vi "main.vi"() -> ()   [LabVIEW 2018]
uses:
  project/type defs/test keypad luster.ctl
  <vilib>/Instr/_visa.llb/VISA Flush IO Buffer Mask.ctl
  <vilib>/Instr/_visa.llb/VISA Configure Serial Port (Instr).vi
  <vilib>/NI/Modbus Library/API/Wrapper/Create Serial Master.vi
  global variables/offset.vi
  type defs/Pelco_D_cmd.vi
  <vilib>/NI/Modbus Library/API/Master/Modbus Master.lvclass
  <vilib>/NI/Modbus Library/API/Wrapper/API Main.lvlib
panel:
  out "Remote TILT":dbl format="%#_6f"
  out "Remote PAN":dbl format="%#_6f"
  in  "Client Closed":string="The client VI closed the connection."
  out "tic":u32
  out "Reset status":bool
  in  "enable":bool=TRUE
  out "tilt":dbl
  out "pan":dbl
  in  "pan_right_limit(-10) 2":dbl=-20.0
  in  "pan left_limit(20) 2":dbl=20.0
  in  "tilt_down_limit(-10)":dbl=-10.0
  in  "tilt_up_limit(20)":dbl=20.0
  in  "delta tilt/sec":dbl=0.1 format="%#.13f"
  in  "delta pan/sec":dbl=0.1 format="%#.13f"
  out "launcher.compass":dbl format="%.1f"
  out "launcher.tilt":dbl format="%.1f"
  out "launcher.pan":dbl format="%.1f"
  out "magnification":string
  in  "get magnification":bool
  in  "cam default":bool
  out "Lancher's Parameters":i16[](array[numeric])
  in  "reset":bool
  out "Sync Status":bool
  out "keypad cmd":string
  out "CAM.tilt":dbl format="%#.2g"
  out "Cam,pan":dbl format="%.2f"
  out "cmd from keypad":string[](array[string])
  out "ressponse tilt":string
  in  "read tilt":bool
  out "ressponse pan":string
  in  "read pan":bool
  in  "close com":bool
  in  "open com":bool
  in  "stop":bool
  in  "VISA resource name":refnum<visa-resource-name>="COM6"
  # "Launcher"
  # "Camera"
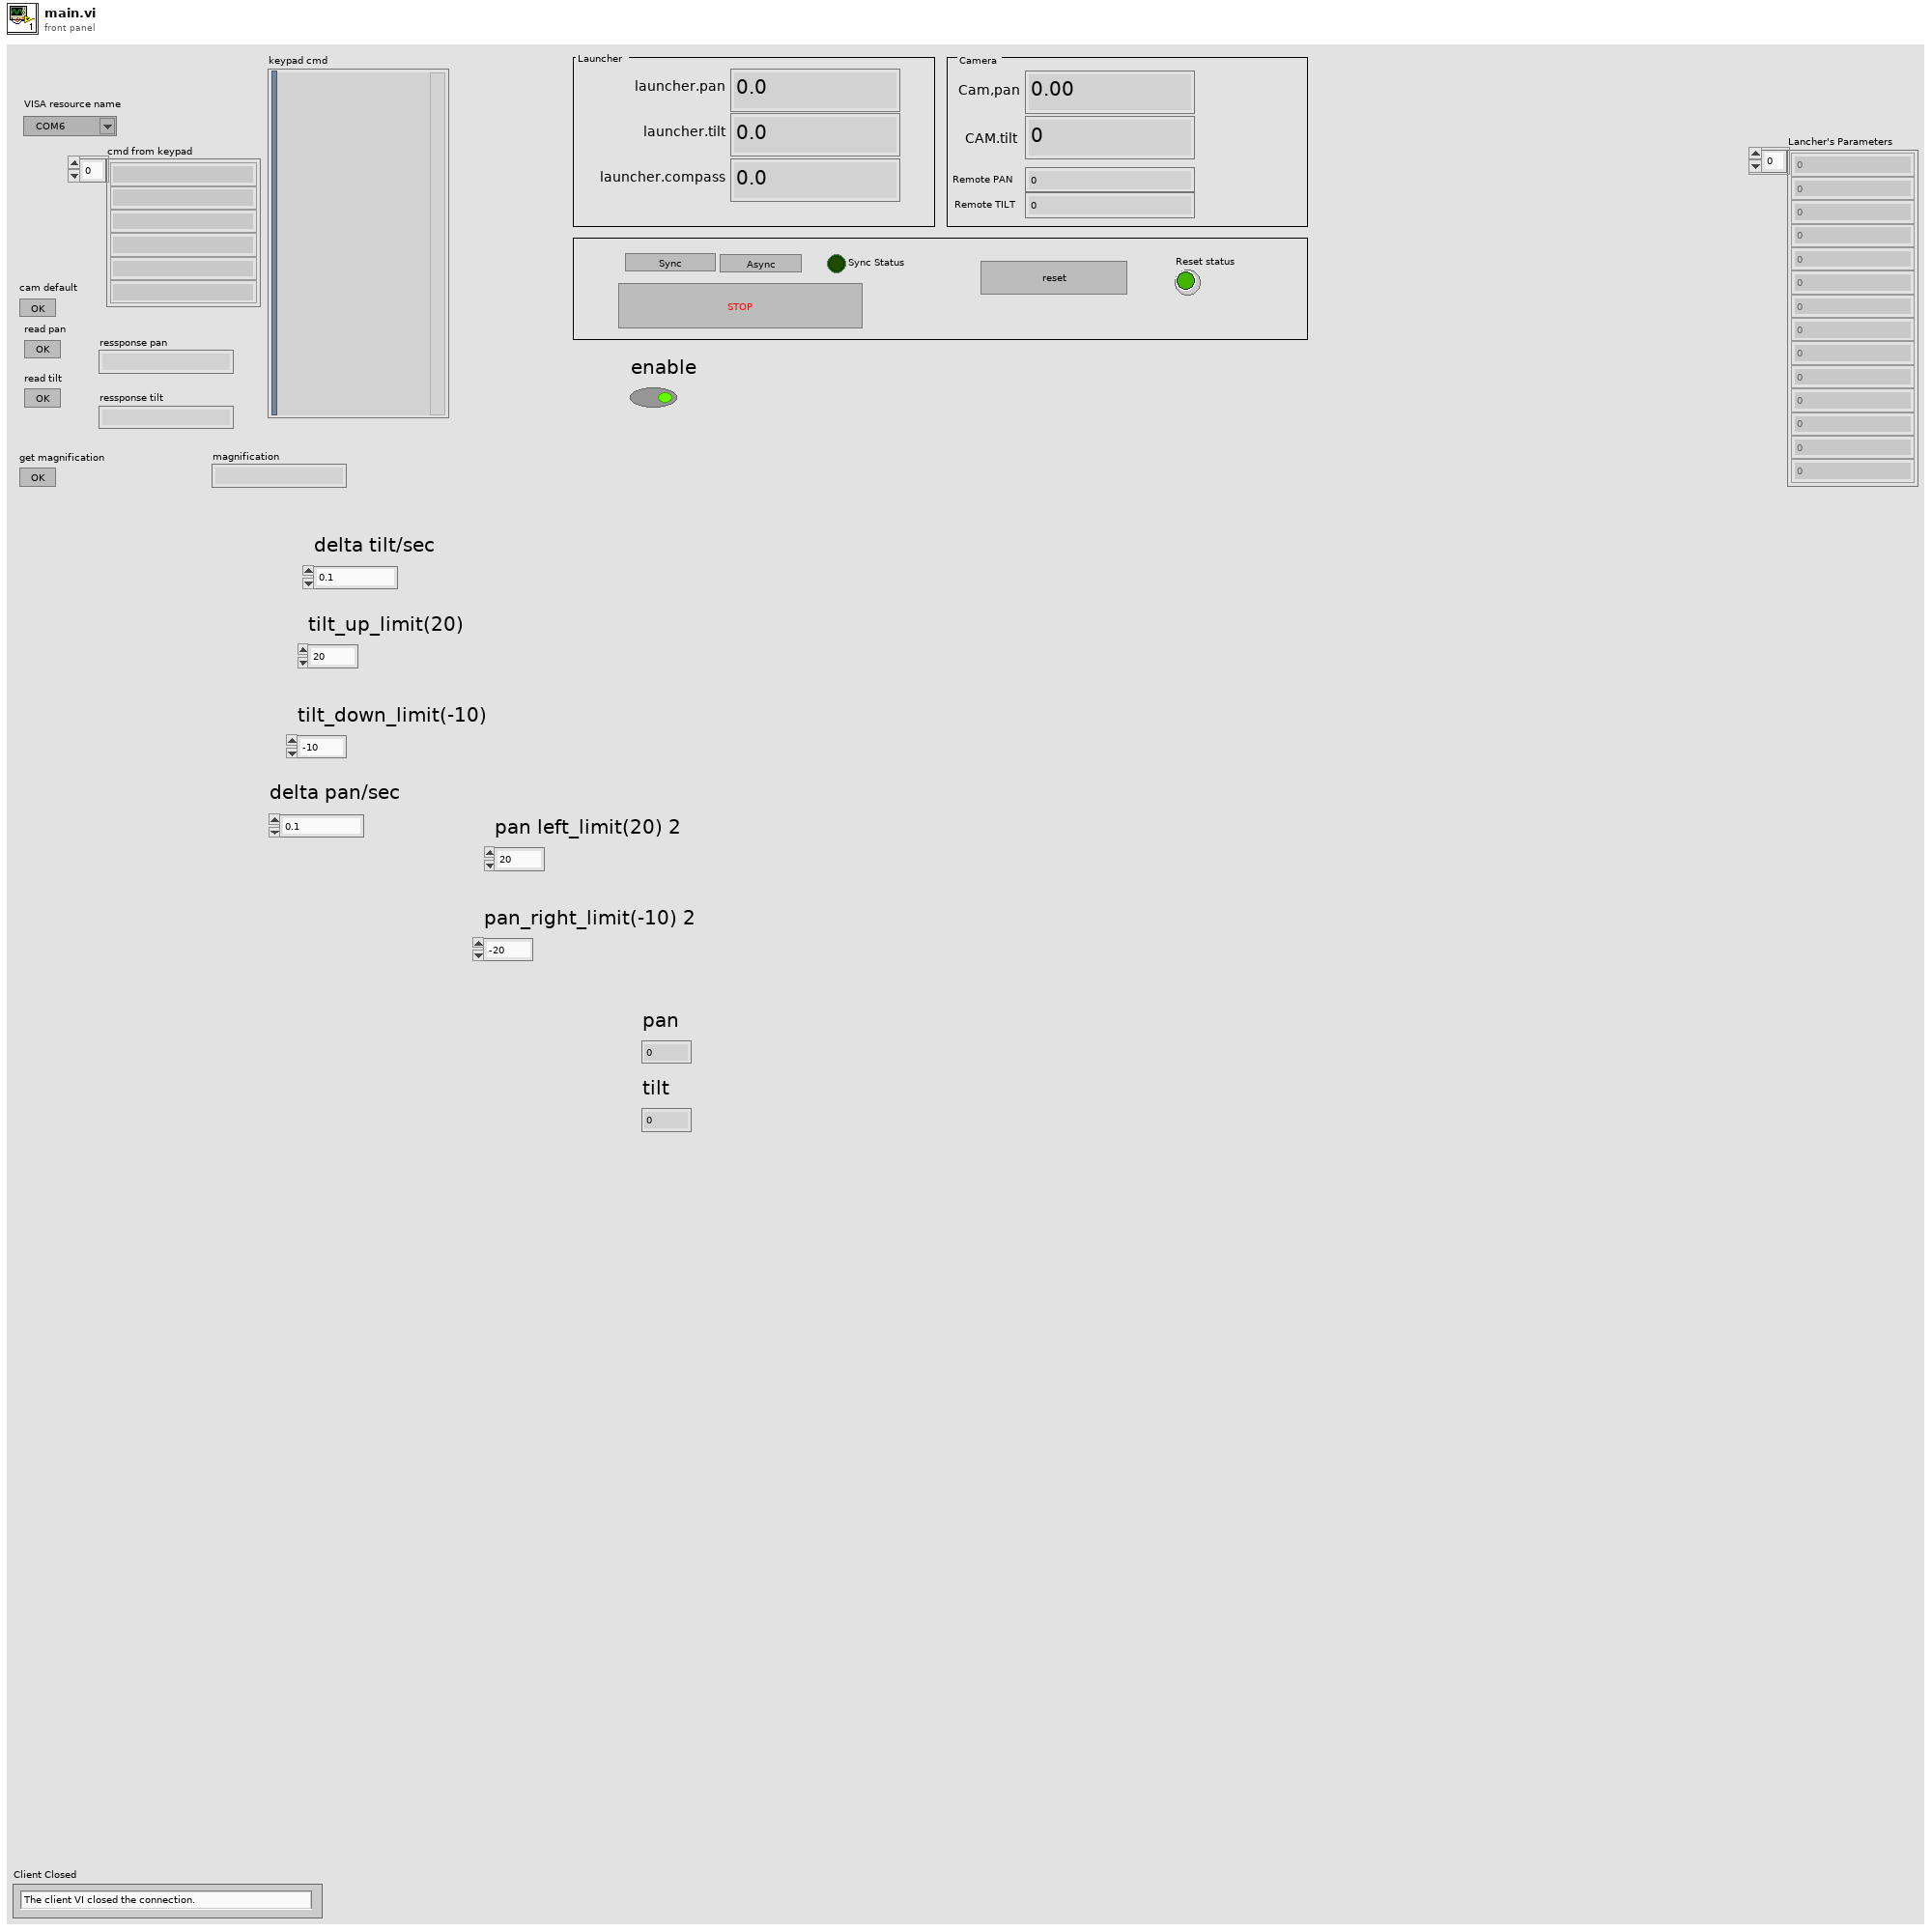
[diagram p1: front panel]
types:
  T1 = cluster{"launcher_pan":i16, "launcher_tilt":i16, "launcher_pan_leftLimit":i16, "launcher_pan_rightLimit":i16, "launcher_tilt_downLimit":i16, "launcher_tilt_upLimit":i16, "launcher_PLClink":i16, "launcher_PLCstatus":i16, "CAM_pan":i16, "CAM_tilt":i16}
  T2 = cluster{"VISA resource name":refnum<visa-resource-name>}
  T3 = typedef "test keypad luster.ctl" = cluster{"cmd":string, "keypad cmd":variant}
  T4 = cluster{"quit":refnum<user-event>, "read tilt":refnum<user-event>, "read pan":refnum<user-event>}
  T5 = typedef "VISA Flush IO Buffer Mask.ctl" = u16
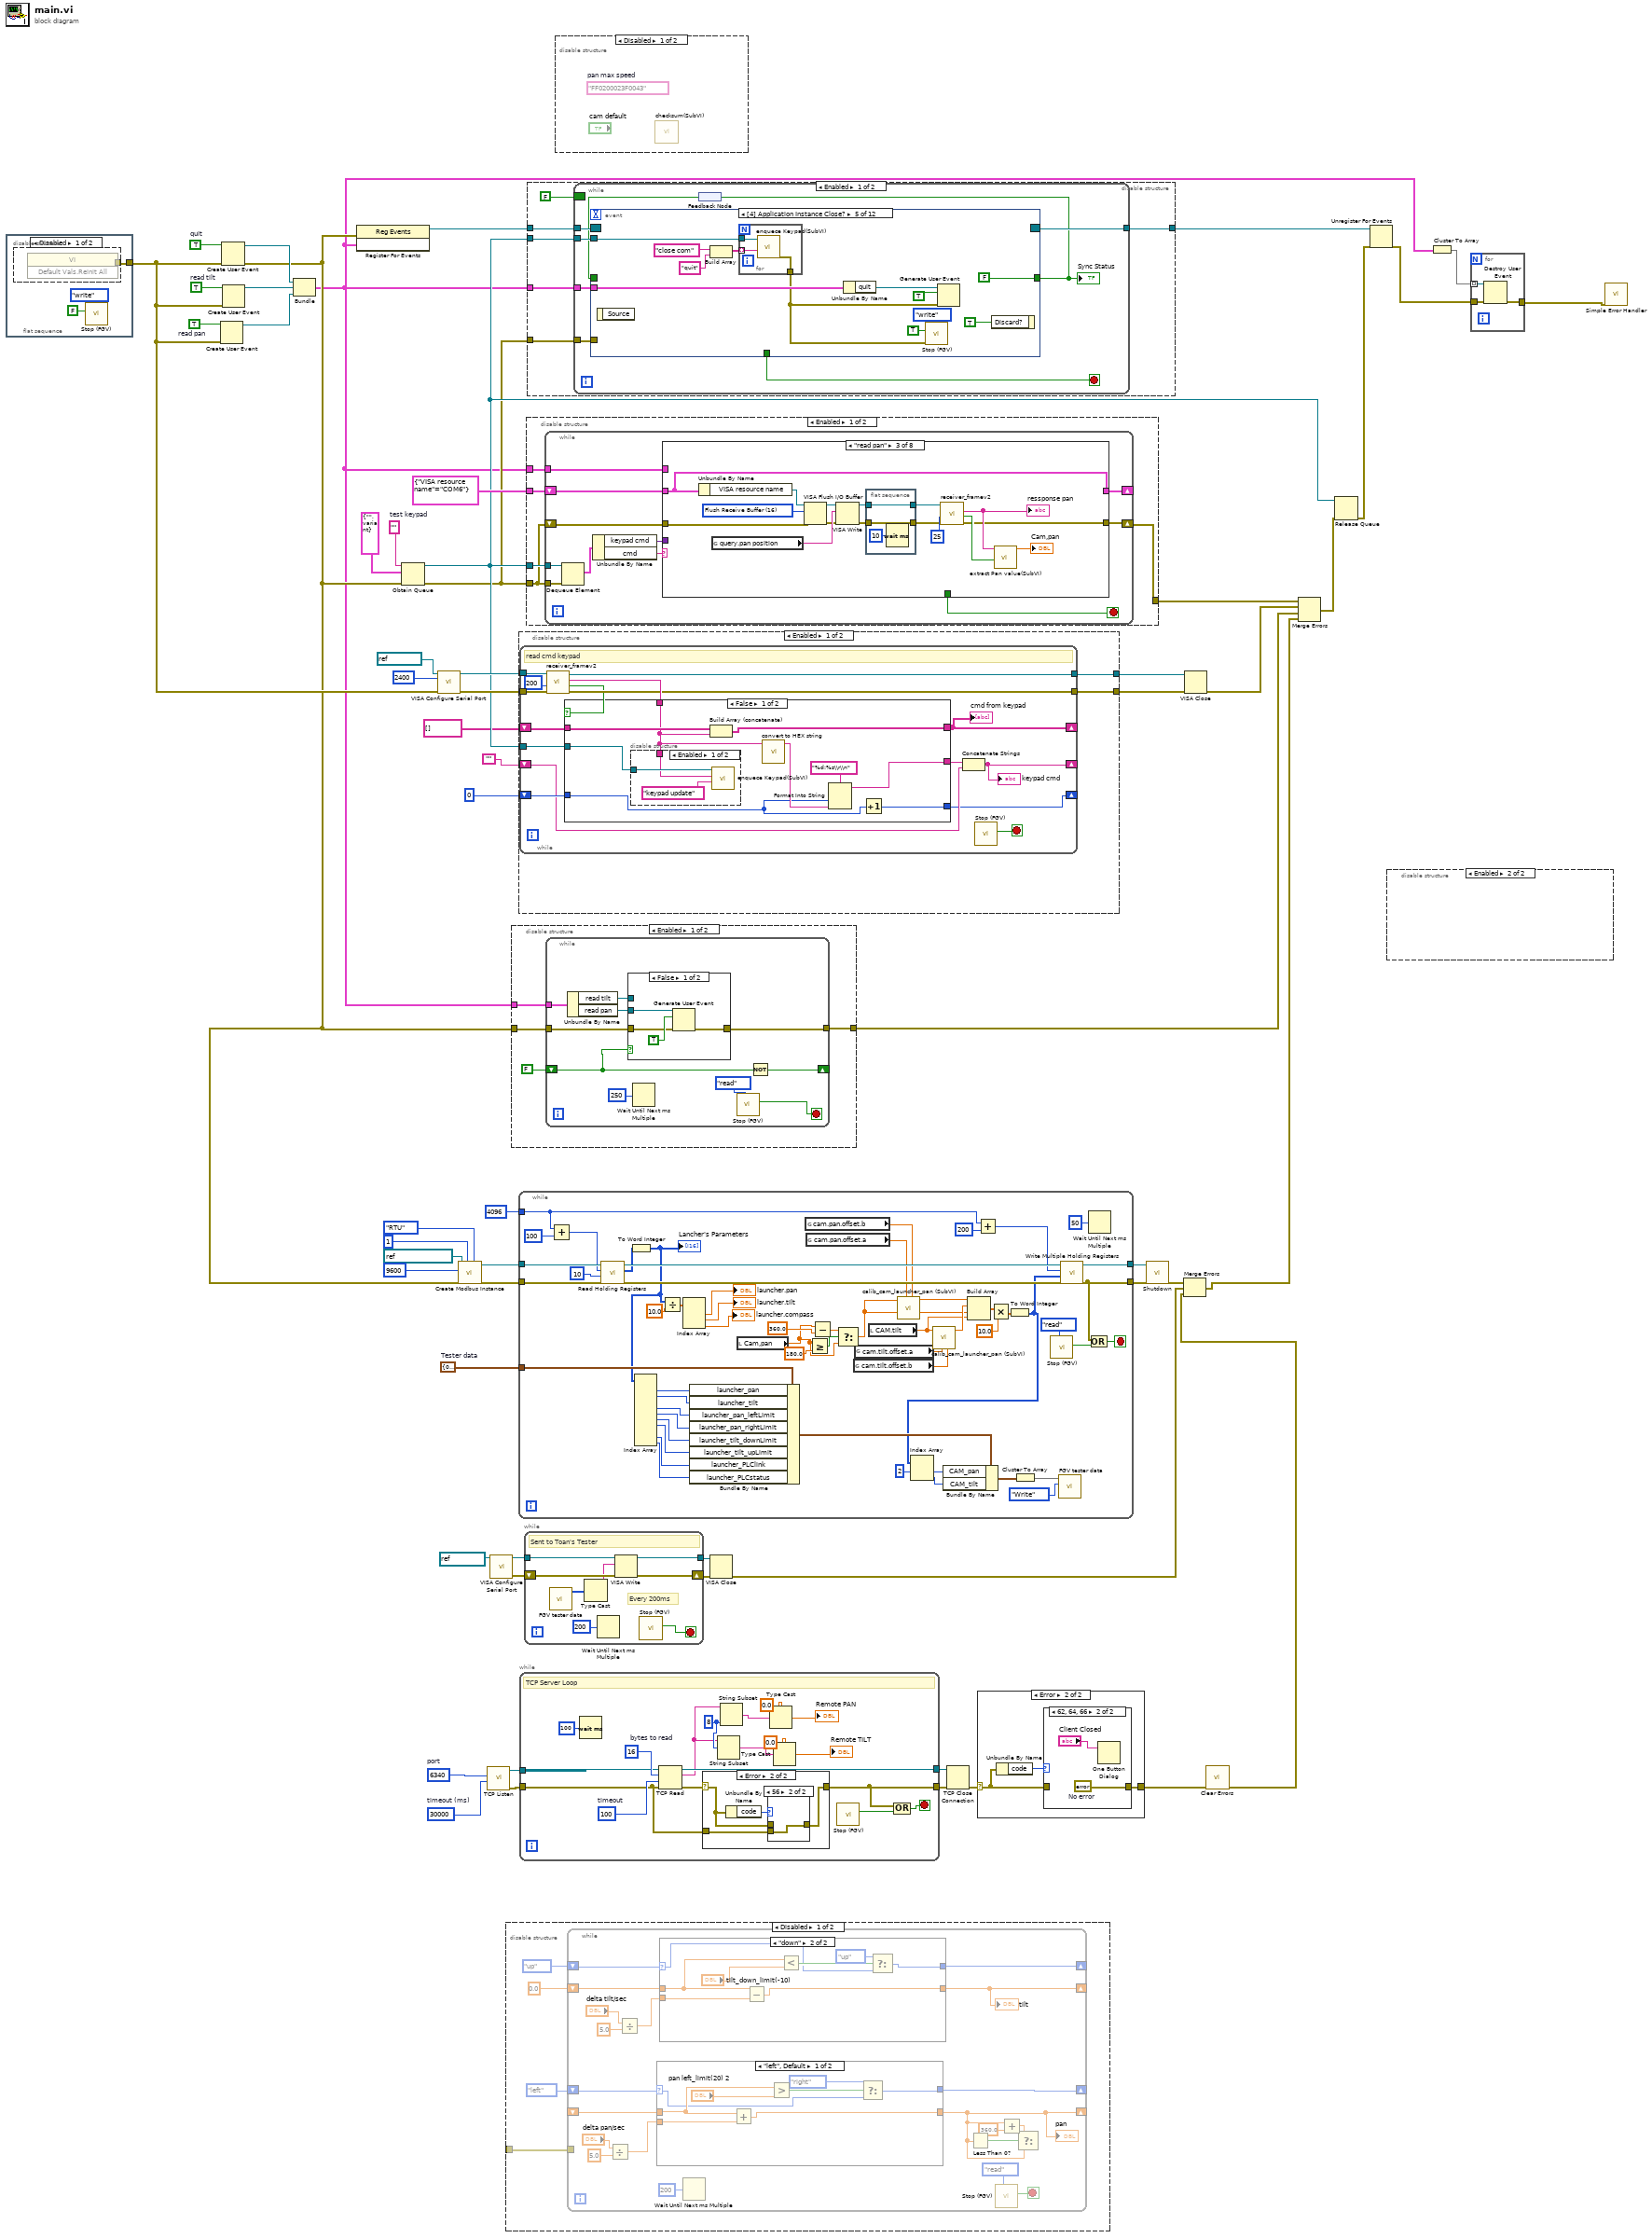
[diagram p0: block diagram]
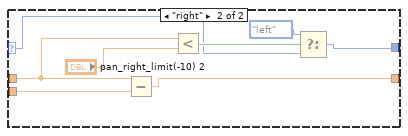
[diagram p7: hidden frame]
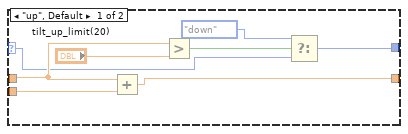
[diagram p8: hidden frame]
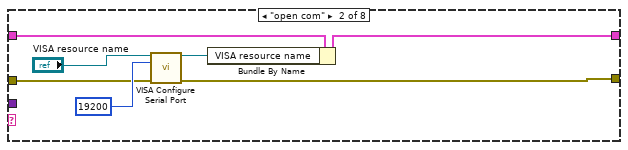
[diagram p11: hidden frame]
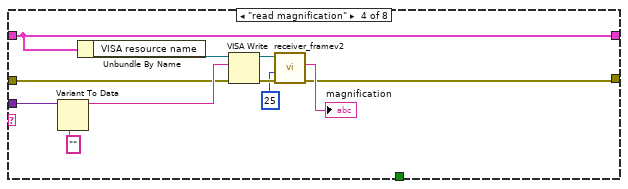
[diagram p12: hidden frame]
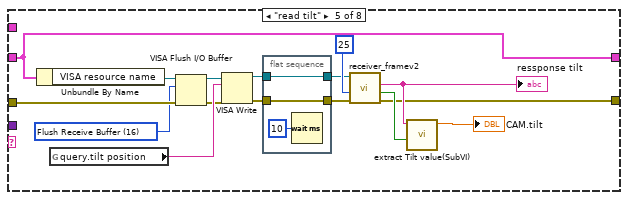
[diagram p13: hidden frame]
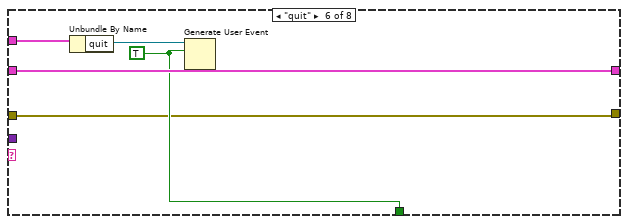
[diagram p14: hidden frame]
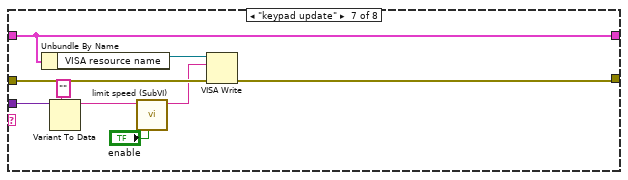
[diagram p15: hidden frame]
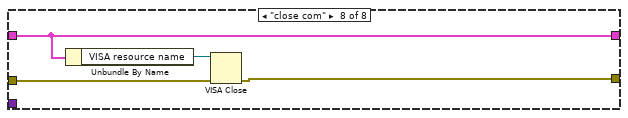
[diagram p16: hidden frame]
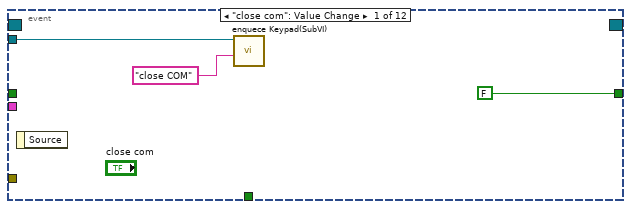
[diagram p18: hidden frame]
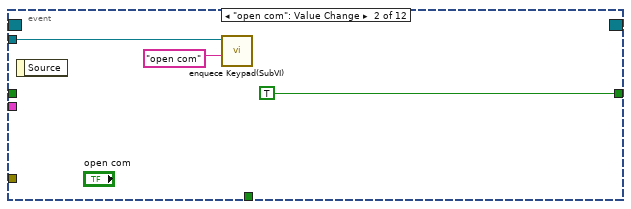
[diagram p19: hidden frame]
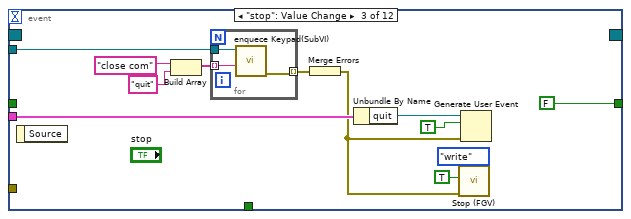
[diagram p20: hidden frame]
diagram:
  w18 = T1 {"launcher_pan"=0, "launcher_tilt"=0, "launcher_pan_leftLimit"=0, "launcher_pan_rightLimit"=0, "launcher_tilt_downLimit"=0, "launcher_tilt_upLimit"=0, "launcher_PLClink"=0, "launcher_PLCstatus"=0, "CAM_pan"=0, "CAM_tilt"=0}  # Tester data
  w3 = u16 6340  # port
  w4 = 30000  # timeout (ms)
  w44 = TRUE  # read pan
  w45 = TRUE  # read tilt
  w59 = TRUE  # quit
  w60 = ""  # test keypad
  n1 = flat-sequence {
    tunnel: [w63] -> w38
    frame #0 {
      n2 = disable-structure shown="Disabled" {
        disable-tunnel: [w64 _] -> w63
        frame Disabled {
          n3 = invoke class="VI" method="Default Vals.Reinit All"() -> (error out=w64:errorcluster)  [unwired: 3 in, 2 out]
        }
        frame Enabled {
        }
      }
      n4 = call "Stop (FGV).vi"("Enum(read)"=enum16{"write", "read"}."write" ("Enum"), "Stop in"=FALSE ("Boolean")) -> ()  [unwired: 8 in, 2 out]
    }
  }
  n5 = Create User Event(user event datatype=w44, error in=w38) -> (user event=w41:refnum<user-event>)  [unwired: 1 out]
  n6 = Create User Event(user event datatype=w59, error in=w38) -> (user event=w43:refnum<user-event>, error out=w30:errorcluster)
  n7 = Create User Event(user event datatype=w45, error in=w38) -> (user event=w42:refnum<user-event>)  [unwired: 1 out]
  n8 = Bundle("quit"=w43, "read tilt"=w42, "read pan"=w41) -> (w29:T4)  [unwired: 1 in]
  n9 = register-events(error in=w30, w29) -> (reference out=w58:refnum<event-registration>)  [unwired: 1 in, 1 out]
  n10 = Obtain Queue(name (unnamed)=w60, element data type=T3 {"cmd"="", "keypad cmd"=variant(refnum<visa-resource-name> "")}, error in (no error)=w30) -> (queue out=w47:refnum<queue>, error out=w33:errorcluster)  [unwired: 2 in, 1 out]
  n11 = call-poly "VISA Configure Serial Port"("VISA resource name"=refnum<visa-resource-name> "COM5", "baud rate (9600)"=u32 2400, "error in (no error)"=w38) -> ("VISA resource name out"=w52:refnum<visa-resource-name>, "error out"=w51:errorcluster)  [unwired: 11 in]
  n12 = call-poly <vilib>:"Create Modbus Instance.vi"("serial type"=enum16{"RTU", "ASCII"}."RTU", "unit ID"=u8 1, "error in"=w30, "baud rate"=u32 9600, "VISA resource name"=refnum<visa-resource-name> "COM1") -> ("error out"=w21:errorcluster, "serial master instance"=w22:refnum<class "Modbus Master.lvclass">)  [unwired: 5 in]
  n13 = call <vilib>:"TCP Listen.vi"("timeout ms (wait forever: -1)"=w4, "port"=w3) -> ("error out"=w5:errorcluster, "connection ID"=w6:refnum<k5>)  [unwired: 5 in, 3 out]
  n14 = call-poly "VISA Configure Serial Port"("VISA resource name"=refnum<visa-resource-name> "COM8") -> ("VISA resource name out"=w16:refnum<visa-resource-name>, "error out"=w15:errorcluster)  [unwired: 13 in]
  n15 = disable-structure shown="Disabled" {
    disable-tunnel: _ -> [w65 _]
    frame Disabled {
      n16 = while {
        shift-right: [w80] -> _
        shift-left: 0.0 -> [w84]
        shift-right: [w75] -> _
        shift-left: _ -> [w82]
        shift-right: [w83] -> _
        shift-left: enum16{"up", "down"}."up" -> [w85]
        shift-right: [w79] -> _
        shift-left: enum16{"left", "right"}."left" -> [w81]
        tunnel: w65 -> [_]
        stop <- w86 stop-if-true
        n17 = Divide(x="delta pan/sec", y=5.0) -> (x/y=w72:dbl)
        n18 = Divide(x="delta tilt/sec", y=5.0) -> (x/y=w69:dbl)
        n19 = case shown="\"left\", Default" w81 {
          selector: w81 -> [w91 w99]
          tunnel: w72 -> [w96 w104]
          tunnel: w82 -> [w94 w102]
          tunnel: [w95 w97] -> w75
          tunnel: [w90 w100] -> w79
          frame "left", Default {
            n20 = Add(x=w94, y=w96) -> (x+y=w95:dbl)
            n21 = Greater?(x=w94, y="pan left_limit(20) 2") -> (0:w92:bool)
            n22 = Select(t=enum16{"left", "right"}."right", s=w92, f=w91) -> (s? t:f=w90:enum16{"left", "right"})
          }
          frame "right" {
            n23 = Subtract(x=w102, y=w104) -> (x-y=w97:dbl)
            n24 = Less?(x=w102, y="pan_right_limit(-10) 2") -> (x < y?=w101:bool)
            n25 = Select(t=enum16{"left", "right"}."left", s=w101, f=w99) -> (s? t:f=w100:enum16{"left", "right"})
          }
        }
        "pan" <- w75
        n26 = case shown="\"down\"" w85 {
          selector: w85 -> [w106 w113]
          tunnel: w69 -> [w112 w120]
          tunnel: w84 -> [w110 w117]
          tunnel: [w111 w119] -> w80
          tunnel: [w105 w115] -> w83
          frame "up", Default {
            n27 = Add(x=w110, y=w112) -> (x+y=w111:dbl)
            n28 = Greater?(x=w110, y="tilt_up_limit(20)") -> (0:w108:bool)
            n29 = Select(t=enum16{"up", "down"}."down", s=w108, f=w106) -> (s? t:f=w105:enum16{"up", "down"})
          }
          frame "down" {
            n30 = Subtract(x=w117, y=w120) -> (x-y=w119:dbl)
            n31 = Less?(x=w117, y="tilt_down_limit(-10)") -> (x < y?=w116:bool)
            n32 = Select(t=enum16{"up", "down"}."up", s=w116, f=w113) -> (s? t:f=w115:enum16{"up", "down"})
          }
        }
        "tilt" <- w80
        n33 = Wait Until Next ms Multiple(millisecond multiple=u32 200) -> ()  [unwired: 1 out]
        n34 = Less Than 0?(x=w75) -> (x < 0?=w78:bool)
        n35 = call "Stop (FGV).vi"("Enum(read)"=enum16{"write", "read"}."read" ("Enum")) -> ("Stop out"=w86:bool)  [unwired: 9 in, 1 out]
        n36 = Add(x=w75, y=360.0) -> (x+y=w76:dbl)
        n37 = Select(t=w76, s=w78, f=w75) -> ()  [unwired: 1 out]
      }
    }
    frame Enabled {
    }
  }
  n38 = disable-structure shown="Enabled" {
    disable-tunnel: w29 -> [w123 _]
    disable-tunnel: w30 -> [w122 w146]
    disable-tunnel: [w121 w146] -> w35
    frame Enabled {
      n39 = while {
        shift-right: [w132] -> _
        shift-left: FALSE -> [w131]
        tunnel: w123 -> [w130]
        tunnel: w122 -> [w129]
        tunnel: [w128] -> w121
        stop <- w133 stop-if-true
        n40 = Unbundle By Name(w130) -> ("read tilt"=w126:refnum<user-event>, "read pan"=w125:refnum<user-event>)
        n41 = case shown="False" w131 {
          tunnel: w126 -> [_ w141]
          tunnel: w125 -> [w138 _]
          tunnel: w129 -> [w136 w140]
          tunnel: [w135 w139] -> w128
          frame False {
            n42 = Generate User Event(user event=w138, event data cluster=TRUE ("event data"), error in=w136) -> (error out=w135:errorcluster)  [unwired: 1 in, 1 out]
          }
          frame True {
            n43 = disable-structure shown="Enabled" {
              disable-tunnel: w141 -> [w145 _]
              disable-tunnel: w140 -> [w143 _]
              disable-tunnel: [w142 _] -> w139
              frame Enabled {
                n44 = Generate User Event(user event=w145, event data cluster=TRUE ("event data"), error in=w143) -> (error out=w142:errorcluster)  [unwired: 1 in, 1 out]
              }
              frame Disabled {
              }
            }
          }
        }
        n45 = Wait Until Next ms Multiple(millisecond multiple=u32 250) -> ()  [unwired: 1 out]
        n46 = call "Stop (FGV).vi"("Enum(read)"=enum16{"write", "read"}."read" ("Enum")) -> ("Stop out"=w133:bool)  [unwired: 9 in, 1 out]
        n47 = Not(x=w131) -> (.not. x?=w132:bool)
      }
    }
    frame Disabled {
    }
  }
  n48 = disable-structure shown="Enabled" {
    disable-tunnel: w52 -> [w154 w201]
    disable-tunnel: w51 -> [w153 w200]
    disable-tunnel: [w152 w200] -> w50
    disable-tunnel: [w151 w201] -> w49
    disable-tunnel: w47 -> [w150 _]
    disable-tunnel: string[] [] -> [w149 _]
    disable-tunnel: u16 0 -> [w148 _]
    disable-tunnel: "" -> [w147 _]
    frame Enabled {
      n49 = while {
        tunnel: w154 -> [w170]
        tunnel: w153 -> [w169]
        shift-right: [w161] -> _
        shift-left: w149 -> [w167]
        tunnel: [w166] -> w152
        tunnel: [w165] -> w151
        tunnel: w150 -> [w163]
        shift-right: [w155] -> _
        shift-left: w147 -> [w157]
        shift-right: [w156] -> _
        shift-left: w148 -> [w159]
        stop <- w162 stop-if-true
        # "read cmd keypad"
        n50 = call "receiver_framev2.vi"("error in (no error)"=w169, "Timeout(100ms)"=u32 200, "Visa In"=w170) -> ("error out"=w166:errorcluster, "TimeOut?"=w164:bool, "response"=w168:string, "Visa out"=w165:refnum<visa-resource-name>)  [unwired: 5 in]
        n51 = case shown="False" w164 {
          tunnel: w168 -> [w176 _]
          tunnel: w167 -> [w178 w186]
          tunnel: [w177 w186] -> w161
          tunnel: w163 -> [w179 w185]
          tunnel: w159 -> [w172 w184]
          tunnel: [w173 _] -> w158
          tunnel: [w171 w184] -> w156
          frame False {
            n52 = disable-structure shown="Enabled" {
              disable-tunnel: w179 -> [w182 _]
              disable-tunnel: w176 -> [w180 _]
              frame Enabled {
                n53 = call "enquece Keypad(SubVI).vi"("keypad cmd"="keypad update" ("cmd"), "cmd"=w180, "Queue in"=w182) -> ()  [unwired: 7 in, 2 out]
              }
              frame Disabled {
              }
            }
            n54 = Build Array (concatenate)(w178, w176) -> (w177:string[])
            n55 = call "convert to HEX string.vi"("String In(binary)"=w176) -> ("String Out (hexa)"=w174:string)  [unwired: 10 in]
            n56 = Format Into String(format string="%d:%s\\r\\n", w172, w174) -> (resulting string=w173:string)  [unwired: 2 in, 1 out]
            n57 = Increment(x=w172) -> (x+1=w171:u16)
          }
          frame True {
            n58 = local read "Reset status"() -> (w183:bool)
            n59 = case shown="False" w183 {
              tunnel: w185 -> [w191 _]
              frame False {
                w187 = "ÿ\u0002\u0000\u0000\u0000\u0000\u0002"  # stop cmd
                w188 = "keypad update" ("cmd")
                w190 = "ÿ\u0001\u0000\u0000\u0000\u0000\u0001"  # stop cmd
                n60 = call "enquece Keypad(SubVI).vi"("keypad cmd"=w188, "cmd"=w190, "Queue in"=w191) -> ("dup quece"=w189:refnum<queue>)  [unwired: 7 in, 1 out]
                n61 = call "enquece Keypad(SubVI).vi"("keypad cmd"=w188, "cmd"=w187, "Queue in"=w189) -> ()  [unwired: 7 in, 2 out]
              }
              frame True {
                n62 = Tick Count (ms)() -> (millisecond timer value=w199:u32)
                n63 = local read "tic"() -> (w198:u32)
                n64 = Subtract(x=w199, y=w198) -> (x-y=w197:u32)
                n65 = Greater Or Equal?(x=w197, y=u32 7000) -> (x >= y?=w195:bool)
                n66 = Select(t=FALSE, s=w195, f=TRUE) -> (s? t:f=w192:bool)
                n67 = local write "Reset status"(w192) -> ()
              }
            }
          }
        }
        "cmd from keypad" <- w161
        n68 = Concatenate Strings(w158, w157) -> (w155:string)
        "keypad cmd" <- w155
        n69 = call "Stop (FGV).vi"() -> ("Stop out"=w162:bool)  [unwired: 10 in, 1 out]
      }
    }
    frame Disabled {
    }
  }
  n70 = while {
    tunnel: u16 4096 -> [w250]
    tunnel: w22 -> [w256]
    tunnel: w21 -> [w252]
    tunnel: [w242] -> w19
    tunnel: [w244] -> w20
    tunnel: w18 -> [w220]
    stop <- w240 stop-if-true
    n71 = Add(x=w250, y=u16 100) -> (x+y=w254:u16)
    n72 = call-dynamic "Read Holding Registers.vi"("error in"=w252, "number of inputs"=u16 10, "starting address"=w254, "Modbus master in"=w256) -> ("error out"=w245:errorcluster, "register values"=w239:u16[], "Modbus master out"=w247:refnum<class "Modbus Master.lvclass">)  [unwired: 5 in]
    n73 = To Word Integer(number=w239) -> (16bit integer=w218:i16[])
    "Lancher's Parameters" <- w218
    n74 = Index Array(array=w218) -> (element #1=w217:i16, element #2=w216:i16, element #4=w215:i16, element #5=w214:i16, element #6=w213:i16, element #7=w212:i16, element #9=w211:i16, element #10=w210:i16)  [unwired: 10 in, 2 out]
    n75 = Divide(x=w218, y=10.0) -> (x/y=w235:dbl[])
    n76 = Index Array(array=w235) -> (element #1=→"launcher.pan":dbl, element #2=→"launcher.tilt":dbl, element #3=→"launcher.compass":dbl)  [unwired: 3 in]
    n77 = Bundle By Name(cluster=w220, "launcher_pan"=w217, "launcher_tilt"=w216, "launcher_pan_leftLimit"=w215, "launcher_pan_rightLimit"=w214, "launcher_tilt_downLimit"=w213, "launcher_tilt_upLimit"=w212, "launcher_PLClink"=w211, "launcher_PLCstatus"=w210) -> (w209:T1)
    n78 = local read "Cam,pan"() -> (w229:dbl)
    n79 = global read "offset.vi" "cam.pan.offset.b"() -> (w223:dbl)
    n80 = global read "offset.vi" "cam.pan.offset.a"() -> (w224:dbl)
    n81 = Greater Or Equal?(x=w229, y=180.0) -> (x >= y?=w232:bool)
    n82 = Subtract(x=w229, y=360.0) -> (x-y=w231:dbl)
    n83 = Select(t=w231, s=w232, f=w229) -> (s? t:f=w226:dbl)
    n84 = global read "offset.vi" "cam.tilt.offset.b"() -> (w221:dbl)
    n85 = global read "offset.vi" "cam.tilt.offset.a"() -> (w222:dbl)
    n86 = local read "CAM.tilt"() -> (w225:dbl)
    n87 = call "calib_cam_launcher_pan (SubVI).vi"("b"=w223, "a"=w224, "x"=w226) -> ("y"=w228:dbl)  [unwired: 8 in]
    n88 = call "calib_cam_launcher_pan (SubVI).vi"("b"=w221, "a"=w222, "x"=w225) -> ("y"=w227:dbl)  [unwired: 8 in]
    n89 = Build Array(w228, w227, w226, w225) -> (w249:dbl[])
    n90 = Add(x=w250, y=u16 200) -> (x+y=w246:u16)
    n91 = Multiply(x=w249, y=10.0) -> (x*y=w219:dbl[])
    n92 = To Word Integer(number=w219) -> (16bit integer=w208:i16[])
    n93 = Index Array(array=w208, index #1=2 ("index")) -> (element #1=w206:i16, element #2=w205:i16)  [unwired: 1 in]
    n94 = Bundle By Name(cluster=w209, "CAM_pan"=w206, "CAM_tilt"=w205) -> (w203:T1)
    n95 = Cluster To Array(cluster=w203) -> (array=w202:i16[])
    n96 = call "Stop (FGV).vi"("Enum(read)"=enum16{"write", "read"}."read" ("Enum")) -> ("Stop out"=w241:bool)  [unwired: 9 in, 1 out]
    n97 = call "FGV tester data.vi"("Enum(read)"=enum16{"Write", "Read"}."Write" ("Enum"), "data in"=w202) -> ()  [unwired: 9 in, 1 out]
    n98 = call-dynamic "Write Multiple Holding Registers.vi"("error in"=w245, "registers to write"=w208, "starting address"=w246, "Modbus master in"=w247) -> ("error out"=w242:errorcluster, "Modbus master out"=w244:refnum<class "Modbus Master.lvclass">)  [unwired: 6 in]
    n99 = Or(x=w242, y=w241) -> (x .or. y?=w240:bool)
    n100 = Wait Until Next ms Multiple(millisecond multiple=u32 50) -> ()  [unwired: 1 out]
  }
  n101 = while {
    tunnel: [w269] -> w8
    tunnel: [w272] -> w9
    tunnel: w6 -> [w268]
    tunnel: w5 -> [w267]
    stop <- w274 stop-if-true
    w263 = 8 ("length (rest)")
    w271 = 100  # timeout
    w273 = 16  # bytes to read
    # "TCP Server Loop"
    n102 = Wait (ms)(milliseconds to wait=u32 100) -> ()  [unwired: 1 out]
    n103 = TCP Read(connection ID=w268, bytes to read=w273, error in (no error)=w267, 9:w271) -> (connection ID out=w272:refnum<k5>, data out=w258:string, error out=w270:errorcluster)  [unwired: 1 out]
    n104 = case shown="Error" w270 {
      selector: w270 -> [w276 w279]
      tunnel: [w276 w277] -> w269
      tunnel: w267 -> [_ w278]
      frame No Error {
      }
      frame Error {
        n105 = Unbundle By Name(w279) -> ("code"=w280:i32)
        n106 = case shown="56" w280 {
          tunnel: w279 -> [w281 _]
          tunnel: w278 -> [_ w282]
          tunnel: [w281 w282] -> w277
          frame Default {
          }
          frame 56 {
          }
        }
      }
    }
    n107 = String Subset(string=w258, offset (0)=w263) -> (substring=w261:string)  [unwired: 1 in]
    n108 = String Subset(string=w258, length (rest)=w263) -> (substring=w265:string)  [unwired: 1 in]
    n109 = Type Cast(type=0.0, x=w265) -> (*(type *) &x=→"Remote PAN":dbl)
    n110 = Type Cast(type=0.0, x=w261) -> (*(type *) &x=→"Remote TILT":dbl)
    n111 = call "Stop (FGV).vi"() -> ("Stop out"=w259:bool)  [unwired: 10 in, 1 out]
    n112 = Compound Arithmetic op=OR(w269, w259) -> (w274:bool)
  }
  n113 = while {
    tunnel: w16 -> [w290]
    shift-right: [w287] -> w14
    shift-left: w15 -> [w289]
    tunnel: [w286] -> w13
    stop <- w288 stop-if-true
    # "Every 200ms"
    # "Sent to Toan's Tester"
    n114 = call "FGV tester data.vi"() -> ("data in 2"=w284:i16[])  [unwired: 11 in]
    n115 = Type Cast(x=w284) -> (*(type *) &x=w283:string)  [unwired: 1 in]
    n116 = Wait Until Next ms Multiple(millisecond multiple=u32 200) -> ()  [unwired: 1 out]
    n117 = VISA Write(VISA resource name=w290, write buffer=w283, error in (no error)=w289) -> (VISA resource name out=w286:refnum<visa-resource-name>, error out=w287:errorcluster)  [unwired: 1 out]
    n118 = call "Stop (FGV).vi"() -> ("Stop out"=w288:bool)  [unwired: 10 in, 1 out]
  }
  n119 = disable-structure shown="Enabled" {
    disable-tunnel: T2 {"VISA resource name"="COM6"} -> [w295 _]
    disable-tunnel: w47 -> [w294 _]
    disable-tunnel: w29 -> [w293 _]
    disable-tunnel: w33 -> [w292 w383]
    disable-tunnel: [w291 w383] -> w32
    frame Enabled {
      n120 = while {
        tunnel: w294 -> [w305]
        tunnel: w292 -> [w306]
        tunnel: w293 -> [w301]
        shift-right: [w302] -> _
        shift-left: w295 -> [w303]
        shift-right: [w296] -> w291
        shift-left: w292 -> [w297]
        stop <- w300 stop-if-true
        n121 = Dequeue Element(queue=w305, error in (no error)=w306) -> (element=w299:T3)  [unwired: 1 in, 3 out]
        n122 = Unbundle By Name(w299) -> ("keypad cmd"=w298:variant, "cmd"=w304:string)
        n123 = case shown="\"read pan\"" w304 {
          tunnel: w303 -> [w308 w312 w331 w340 w361 w369 w375 w381]
          tunnel: [w308 w311 w331 w340 w361 w369 w375 w381] -> w302
          tunnel: w301 -> [_ _ _ _ _ w367 _ _]
          tunnel: [_ _ _ _ _ w368 _ _] -> w300
          tunnel: w298 -> [_ _ _ w339 _ _ w377 _]
          tunnel: w297 -> [w307 w310 w322 w336 w353 w365 w374 w380]
          tunnel: [w307 w309 w326 w335 w352 w365 w373 w379] -> w296
          frame "False", Default {
          }
          frame "open com" {
            n124 = call-poly "VISA Configure Serial Port"("VISA resource name"="VISA resource name", "baud rate (9600)"=u32 19200, "error in (no error)"=w310) -> ("VISA resource name out"=w313:refnum<visa-resource-name>, "error out"=w309:errorcluster)  [unwired: 11 in]
            n125 = Bundle By Name(cluster=w312, "VISA resource name"=w313) -> (w311:T2)
          }
          frame "read pan" {
            w325 = T5 16 items=["Flush Receive Buffer"=16, "Write Transmit Buffer to Device"=32, "Flush Receive Buffer (No I/O)"=64, "Flush Transmit Buffer"=128] ("Mask")
            n126 = Unbundle By Name(w331) -> ("VISA resource name"=w324:refnum<visa-resource-name>)
            n127 = global read "Pelco_D_cmd.vi" "query.pan position"() -> (w327:string)
            n128 = VISA Flush I/O Buffer(VISA resource name=w324, mask (16)=w325, error in (no error)=w322) -> (VISA resource name out=w323:refnum<visa-resource-name>, error out=w321:errorcluster)
            n129 = VISA Write(VISA resource name=w323, write buffer=w327, error in (no error)=w321) -> (VISA resource name out=w319:refnum<visa-resource-name>, error out=w317:errorcluster)  [unwired: 1 out]
            n130 = flat-sequence {
              tunnel: [w334] -> w320
              tunnel: w319 -> [w334]
              tunnel: [w333] -> w318
              tunnel: w317 -> [w333]
              frame #0 {
                n131 = Wait (ms)(milliseconds to wait=u32 10) -> ()  [unwired: 1 out]
              }
            }
            n132 = call "receiver_framev2.vi"("error in (no error)"=w318, "Timeout(100ms)"=u32 25, "Visa In"=w320) -> ("error out"=w326:errorcluster, "TimeOut?"=w329:bool, "response"=w330:string)  [unwired: 5 in, 1 out]
            "ressponse pan" <- w330
            n133 = call "extract Pan value(SubVI).vi"("TimeOut"=w329, "response"=w330) -> ("pan angle"=→"Cam,pan":dbl)  [unwired: 8 in, 1 out]
          }
          frame "read magnification" {
            n134 = Variant To Data(type="", Variant=w339) -> (data=w337:string)  [unwired: 1 in, 1 out]
            n135 = Unbundle By Name(w340) -> ("VISA resource name"=w345:refnum<visa-resource-name>)
            n136 = VISA Write(VISA resource name=w345, write buffer=w337, error in (no error)=w336) -> (VISA resource name out=w344:refnum<visa-resource-name>, error out=w343:errorcluster)  [unwired: 1 out]
            n137 = call "receiver_framev2.vi"("error in (no error)"=w343, "Timeout(100ms)"=u32 25, "Visa In"=w344) -> ("error out"=w335:errorcluster, "response"=→"magnification":string)  [unwired: 5 in, 2 out]
          }
          frame "read tilt" {
            w351 = T5 16 items=["Flush Receive Buffer"=16, "Write Transmit Buffer to Device"=32, "Flush Receive Buffer (No I/O)"=64, "Flush Transmit Buffer"=128] ("Mask")
            n138 = Unbundle By Name(w361) -> ("VISA resource name"=w356:refnum<visa-resource-name>)
            n139 = global read "Pelco_D_cmd.vi" "query.tilt position"() -> (w357:string)
            n140 = VISA Flush I/O Buffer(VISA resource name=w356, mask (16)=w351, error in (no error)=w353) -> (VISA resource name out=w355:refnum<visa-resource-name>, error out=w354:errorcluster)
            n141 = VISA Write(VISA resource name=w355, write buffer=w357, error in (no error)=w354) -> (VISA resource name out=w349:refnum<visa-resource-name>, error out=w347:errorcluster)  [unwired: 1 out]
            n142 = flat-sequence {
              tunnel: [w363] -> w350
              tunnel: w349 -> [w363]
              tunnel: [w362] -> w348
              tunnel: w347 -> [w362]
              frame #0 {
                n143 = Wait (ms)(milliseconds to wait=u32 10) -> ()  [unwired: 1 out]
              }
            }
            n144 = call "receiver_framev2.vi"("error in (no error)"=w348, "Timeout(100ms)"=u32 25, "Visa In"=w350) -> ("error out"=w352:errorcluster, "TimeOut?"=w359:bool, "response"=w360:string)  [unwired: 5 in, 1 out]
            "ressponse tilt" <- w360
            n145 = call "extract Tilt value(SubVI).vi"("Time out?"=w359, "Pelco-D response"=w360) -> ("tilt1"=→"CAM.tilt":dbl)  [unwired: 8 in, 1 out]
          }
          frame "quit" {
            w368 = TRUE ("event data")
            n146 = Unbundle By Name(w367) -> ("quit"=w366:refnum<user-event>)
            n147 = Generate User Event(user event=w366, event data cluster=w368) -> ()  [unwired: 2 in, 2 out]
          }
          frame "keypad update" {
            n148 = Unbundle By Name(w375) -> ("VISA resource name"=w376:refnum<visa-resource-name>)
            n149 = Variant To Data(type="", Variant=w377) -> (data=w372:string)  [unwired: 1 in, 1 out]
            n150 = call "limit speed (SubVI).vi"("enable"="enable", "keypad cmd"=w372) -> ("keypad cmd  out"=w371:string)  [unwired: 9 in]
            n151 = VISA Write(VISA resource name=w376, write buffer=w371, error in (no error)=w374) -> (error out=w373:errorcluster)  [unwired: 2 out]
          }
          frame "close com" {
            n152 = Unbundle By Name(w381) -> ("VISA resource name"=w382:refnum<visa-resource-name>)
            n153 = VISA Close(VISA resource name=w382, error in (no error)=w380) -> (error out=w379:errorcluster)
          }
        }
      }
    }
    frame Disabled {
    }
  }
  n154 = disable-structure shown="Enabled" {
    disable-tunnel: w58 -> [w389 w478]
    disable-tunnel: [w388 w478] -> w57
    disable-tunnel: w47 -> [w387 _]
    disable-tunnel: w33 -> [w385 _]
    disable-tunnel: w29 -> [w384 _]
    frame Enabled {
      n155 = while {
        tunnel: w387 -> [w395]
        tunnel: w385 -> [w397]
        tunnel: w389 -> [w396]
        tunnel: [w394] -> w388
        border: FALSE -> [_]
        tunnel: w384 -> [w390]
        stop <- w393 stop-if-true
        n156 = feedback #1() -> (w391:bool)
        n157 = event shown="[4] Application Instance Close?" {
          selector: w396 -> [_ _ _ _ _ _ _ _ _ _ _ _]
          dyn-events: [_ _ _ _ _ _ _ _ _ _ _ _] -> w394
          timeout: _ -> [_ _ _ _ _ _ _ _ _ _ _ _]
          tunnel: w397 -> [_ _ _ _ _ _ _ _ _ _ _ _]
          tunnel: w395 -> [w400 w402 w415 w430 w445 _ w452 w456 w457 w462 w470 w476]
          tunnel: [_ _ _ _ _ w450 _ _ _ _ _ _] -> w393
          tunnel: [FALSE TRUE FALSE FALSE FALSE w449 w451 w454 w459 w460 w467 w477] -> w392
          tunnel: w391 -> [_ _ _ _ _ w449 w451 w454 w459 w460 w467 w477]
          tunnel: w390 -> [_ _ w408 w423 w438 _ _ _ _ _ _ _]
          event "close com": Value Change {
            n158 = event-data() -> ()  [unwired: 1 in, 1 out]
            n159 = call "enquece Keypad(SubVI).vi"("keypad cmd"="close COM" ("cmd"), "Queue in"=w400) -> ()  [unwired: 8 in, 2 out]
          }
          event "open com": Value Change {
            n160 = event-data() -> ()  [unwired: 1 in, 1 out]
            n161 = call "enquece Keypad(SubVI).vi"("keypad cmd"="open com" ("element"), "Queue in"=w402) -> ()  [unwired: 8 in, 2 out]
          }
          event "stop": Value Change {
            n162 = event-data() -> ()  [unwired: 1 in, 1 out]
            n163 = Build Array("close com", "quit") -> (w410:string[])
            n164 = for {
              tunnel: w410 -> [w418] mode=indexing
              tunnel: w415 -> [w417]
              tunnel: [w416] -> w405 mode=indexing
              n165 = call "enquece Keypad(SubVI).vi"("keypad cmd"=w418, "Queue in"=w417) -> ("error out"=w416:errorcluster)  [unwired: 8 in, 1 out]
            }
            n166 = Merge Errors(w405) -> (w404:errorcluster)
            n167 = Unbundle By Name(w408) -> ("quit"=w407:refnum<user-event>)
            n168 = call "Stop (FGV).vi"("Enum(read)"=enum16{"write", "read"}."write" ("Enum"), "error in (no error)"=w404, "Stop in"=TRUE ("Boolean")) -> ()  [unwired: 7 in, 2 out]
            n169 = Generate User Event(user event=w407, event data cluster=TRUE, error in=w404) -> ()  [unwired: 1 in, 2 out]
          }
          event Panel Close? {
            n170 = event-data() -> ()  [unwired: 1 in, 4 out]
            n171 = Build Array("close com", "quit") -> (w425:string[])
            n172 = for {
              tunnel: w425 -> [w433] mode=indexing
              tunnel: w430 -> [w432]
              tunnel: [w431] -> w420
              n173 = call "enquece Keypad(SubVI).vi"("keypad cmd"=w433, "Queue in"=w432) -> ("error out"=w431:errorcluster)  [unwired: 8 in, 1 out]
            }
            n174 = Unbundle By Name(w423) -> ("quit"=w422:refnum<user-event>)
            n175 = call "Stop (FGV).vi"("Enum(read)"=enum16{"write", "read"}."write" ("Enum"), "error in (no error)"=w420, "Stop in"=TRUE ("Boolean")) -> ()  [unwired: 7 in, 2 out]
            n176 = Generate User Event(user event=w422, event data cluster=TRUE, error in=w420) -> ()  [unwired: 1 in, 2 out]
            n177 = event-data("Discard?"=TRUE) -> ()  [unwired: 1 in, 1 out]
          }
          event Application Instance Close? {
            n178 = event-data() -> ()  [unwired: 1 in, 1 out]
            n179 = Build Array("close com", "quit") -> (w440:string[])
            n180 = for {
              tunnel: w440 -> [w448] mode=indexing
              tunnel: w445 -> [w447]
              tunnel: [w446] -> w435
              n181 = call "enquece Keypad(SubVI).vi"("keypad cmd"=w448, "Queue in"=w447) -> ("error out"=w446:errorcluster)  [unwired: 8 in, 1 out]
            }
            n182 = Unbundle By Name(w438) -> ("quit"=w437:refnum<user-event>)
            n183 = call "Stop (FGV).vi"("Enum(read)"=enum16{"write", "read"}."write" ("Enum"), "error in (no error)"=w435, "Stop in"=TRUE ("Boolean")) -> ()  [unwired: 7 in, 2 out]
            n184 = Generate User Event(user event=w437, event data cluster=TRUE, error in=w435) -> ()  [unwired: 1 in, 2 out]
            n185 = event-data("Discard?"=TRUE) -> ()  [unwired: 1 in, 1 out]
          }
          event User Event {
            n186 = event-data() -> ("quit"=w450:bool)  [unwired: 1 in]
          }
          event User Event {
            n187 = event-data() -> ()  [unwired: 1 in, 1 out]
            n188 = call "enquece Keypad(SubVI).vi"("keypad cmd"="read pan", "Queue in"=w452) -> ()  [unwired: 8 in, 2 out]
          }
          event "read tilt": Value Change {
            n189 = event-data() -> ()  [unwired: 1 in, 6 out]
            n190 = call "enquece Keypad(SubVI).vi"("keypad cmd"="read tilt" ("cmd"), "Queue in"=w456) -> ()  [unwired: 8 in, 2 out]
          }
          event "read pan": Value Change {
            n191 = event-data() -> ()  [unwired: 1 in, 6 out]
            n192 = call "opposite enquece Keypad(SubVI).vi"("cmd"="read pan", "Queue in"=w457) -> ()  [unwired: 8 in, 2 out]
          }
          event User Event {
            n193 = event-data() -> ()  [unwired: 1 in, 1 out]
            n194 = call "opposite enquece Keypad(SubVI).vi"("cmd"="read tilt", "Queue in"=w462) -> ()  [unwired: 8 in, 2 out]
          }
          event "reset": Value Change {
            n195 = event-data() -> ()  [unwired: 1 in, 4 out]
            n196 = global read "Pelco_D_cmd.vi" "query.set position pan zero"() -> (w466:string)
            n197 = global read "Pelco_D_cmd.vi" "query.set position tilt zero"() -> (w465:string)
            n198 = Build Array(w466, w465) -> (w469:string[])
            n199 = Tick Count (ms)() -> (millisecond timer value=→"tic":u32)
            n200 = for {
              tunnel: w470 -> [w473]
              tunnel: w469 -> [w472] mode=indexing
              tunnel: "keypad update" ("cmd") -> [w471]
              n201 = call "enquece Keypad(SubVI).vi"("keypad cmd"=w471, "cmd"=w472, "Queue in"=w473) -> ()  [unwired: 7 in, 2 out]
            }
            "Reset status" <- TRUE
          }
          event "get magnification": Value Change {
            n202 = event-data() -> ()  [unwired: 1 in, 1 out]
            n203 = global read "Pelco_D_cmd.vi" "query. query magnification"() -> (w475:string)
            n204 = call "enquece Keypad(SubVI).vi"("keypad cmd"="keypad update" ("cmd"), "cmd"=w475, "Queue in"=w476) -> ()  [unwired: 7 in, 2 out]
          }
        }
        "Sync Status" <- w392
        n205 = feedback-in #1(w392) -> ()
      }
    }
    frame Disabled {
    }
  }
  n206 = disable-structure shown="Disabled" {
    frame Disabled {
      (unwired) "FF0200023F0043"  # pan max speed
      n207 = call "checksum(SubVI).vi"() -> ()  [unwired: 11 in, 1 out]
    }
    frame Enabled {
    }
  }
  n208 = VISA Close(VISA resource name=w13, error in (no error)=w14) -> (error out=w12:errorcluster)
  n209 = TCP Close Connection(connection ID=w9, error in (no error)=w8) -> (error out=w7:errorcluster)  [unwired: 2 out]
  n210 = case shown="Error" w7 {
    selector: w7 -> [w479 w481]
    tunnel: [w479 w480] -> w2
    frame No Error {
    }
    frame Error {
      n211 = Unbundle By Name(w481) -> ("code"=w482:i32)
      n212 = case shown="62, 64, 66" w482 {
        tunnel: w481 -> [w483 _]
        tunnel: [w483 w485] -> w480
        frame Default {
        }
        frame 62, 64, 66 {
          w485 = errorcluster {"status"=FALSE, "code"=0, "source"=""}  # No error
          n213 = One Button Dialog(message="Client Closed") -> ()  [unwired: 1 in, 1 out]
        }
      }
    }
  }
  n214 = call-dynamic "Shutdown.vi"("error in"=w19, "Modbus master in"=w20) -> ("error out"=w11:errorcluster)  [unwired: 9 in]
  n215 = VISA Close(VISA resource name=w49, error in (no error)=w50) -> (error out=w34:errorcluster)
  n216 = call <vilib>:"Clear Errors.vi"("error in (no error)"=w2) -> ("error out"=w1:errorcluster)  [unwired: 5 in, 1 out]
  n217 = Merge Errors(w11, w12, w1) -> (w10:errorcluster)
  n218 = Merge Errors(w32, w34, w35, w10) -> (w37:errorcluster)
  n219 = Release Queue(queue=w47, error in (no error)=w37) -> (error out=w46:errorcluster)  [unwired: 1 in, 2 out]
  n220 = Unregister For Events(event registration refnum=w57, error in=w46) -> (error out=w56:errorcluster)
  n221 = disable-structure shown="Enabled" {
    frame Disabled {
      n222 = Unbundle By Name() -> ("VISA resource name"=w486:refnum<visa-resource-name>)  [unwired: 1 in]
      n223 = VISA Close(VISA resource name=w486) -> ()  [unwired: 1 in, 1 out]
    }
    frame Enabled {
    }
  }
  n224 = Cluster To Array(cluster=w29) -> (array=w40:refnum<user-event>[])
  n225 = for {
    tunnel: w56 -> [w489]
    tunnel: w40 -> [w488] mode=indexing
    tunnel: [w487] -> w39
    n226 = Destroy User Event(user event=w488, error in=w489) -> (error out=w487:errorcluster)
  }
  n227 = call <vilib>:"Simple Error Handler.vi"("error in (no error)"=w39) -> ()  [unwired: 4 in, 5 out]
